vi "Compute Tag Angles.vi"(9 "IMU offset":dbl, 10 "tag info":dbl[][](array[numeric]), 11 "located tags":T1(array[cluster])) -> (2 "Vectors":cluster{cluster{"X":dbl, "Y":dbl}[]}[](array[cluster]), 3 "updated tags":T2(array[cluster]))   [LabVIEW 2023]
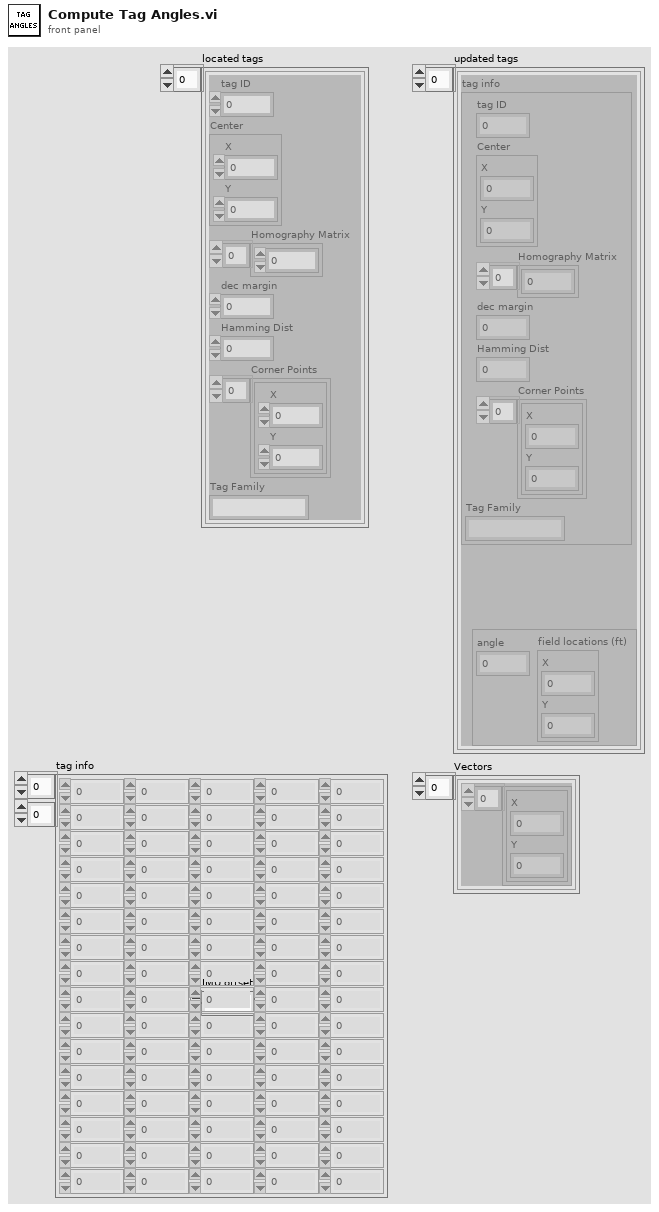
[diagram p1: front panel]
types:
  T1 = cluster{"tag ID":i32, "Center":cluster{"X":dbl, "Y":dbl}, "Homography Matrix":dbl[], "dec margin":dbl, "Hamming Dist":i32, "Corner Points":cluster{"X":dbl, "Y":dbl}[], "Tag Family":string}[]
  T2 = cluster{"tag info":cluster{"tag ID":i32, "Center":cluster{"X":dbl, "Y":dbl}, "Homography Matrix":dbl[], "dec margin":dbl, "Hamming Dist":i32, "Corner Points":cluster{"X":dbl, "Y":dbl}[], "Tag Family":string}, cluster{"angle":dbl, "field locations (ft)":cluster{"X":dbl, "Y":dbl}}}[]
  T3 = cluster{"angle":dbl, "field locations (ft)":cluster{"X":dbl, "Y":dbl}}
  T4 = cluster{"tag info":cluster{"tag ID":i32, "Center":cluster{"X":dbl, "Y":dbl}, "Homography Matrix":dbl[], "dec margin":dbl, "Hamming Dist":i32, "Corner Points":cluster{"X":dbl, "Y":dbl}[], "Tag Family":string}, cluster{"angle":dbl, "field locations (ft)":cluster{"X":dbl, "Y":dbl}}}
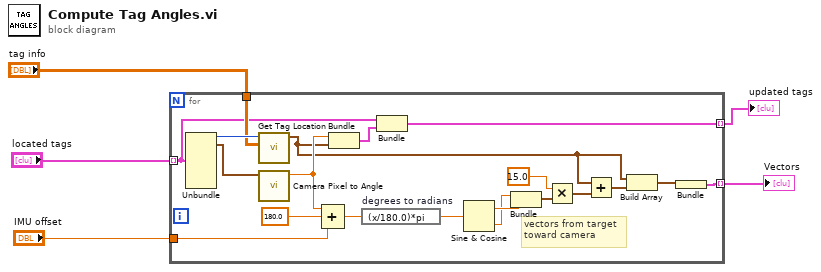
[diagram p0: block diagram]
diagram:
  n1 = for {
    tunnel: "located tags" -> [w22] mode=indexing
    tunnel: "tag info" -> [w24]
    tunnel: [w21] -> w4 mode=indexing
    tunnel: [w9] -> w3 mode=indexing
    tunnel: "IMU offset" -> [w8]
    # "vectors from target\ntoward camera"
    n2 = Unbundle(w22) -> ("tag ID"=w25:i32, "Center"=w20:cluster{"X":dbl, "Y":dbl})  [unwired: 5 out]
    n3 = call "Get Tag Location.vi"("tag info"=w24, "tag ID"=w25) -> ("field locations (ft)"=w6:cluster{"X":dbl, "Y":dbl})  [unwired: 9 in]
    n4 = call "Camera Pixel to Angle.vi"("Point (px)"=w20) -> ("angle"=w7:dbl)  [unwired: 10 in]
    n5 = Compound Arithmetic op=ADD(w7, 180.0 ("y"), w8) -> (w18:dbl)
    n6 = Bundle("angle"=w7, "field locations (ft)"=w6) -> (w23:T3)  [unwired: 1 in]
    n7 = expression code="(x/180.0)*pi" "degrees to radians"(w18) -> (w17:dbl)
    n8 = Bundle("tag info"=w22, w23) -> (w21:T4)  [unwired: 1 in]
    n9 = Sine & Cosine(0:w17) -> (1:w16:dbl, 2:w15:dbl)
    n10 = Bundle(w15, w16) -> (w14:cluster{dbl, dbl})  [unwired: 1 in]
    n11 = Multiply(x=15.0, y=w14) -> (x*y=w13:cluster{dbl, dbl})
    n12 = Add(x=w6, y=w13) -> (x+y=w11:cluster{dbl, dbl})
    n13 = Build Array(w6, w11) -> (w10:cluster{"X":dbl, "Y":dbl}[])
    n14 = Bundle(w10) -> (w9:cluster{cluster{"X":dbl, "Y":dbl}[]})  [unwired: 1 in]
  }
  "updated tags" <- w4
  "Vectors" <- w3
